vi "Build Support lvproj PPLs.vi"(8 "error in":errorcluster, 11 "custom device path":path) -> (0 "error out":errorcluster, 3 "custom device path out":path)   [LabVIEW 2020, in "Template Tool.lvlib"]
uses:
  Template Tool.lvlib
  Template Tool Global.vi
  <vilib>/AppBuilder/AB_API_Simple/NI_App_Builder_API.lvlib
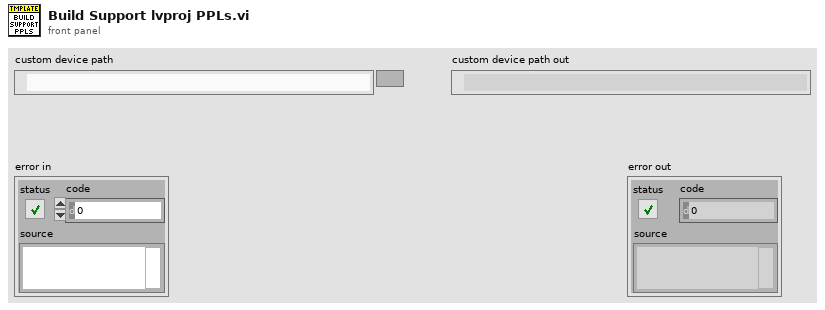
[diagram p1: front panel]
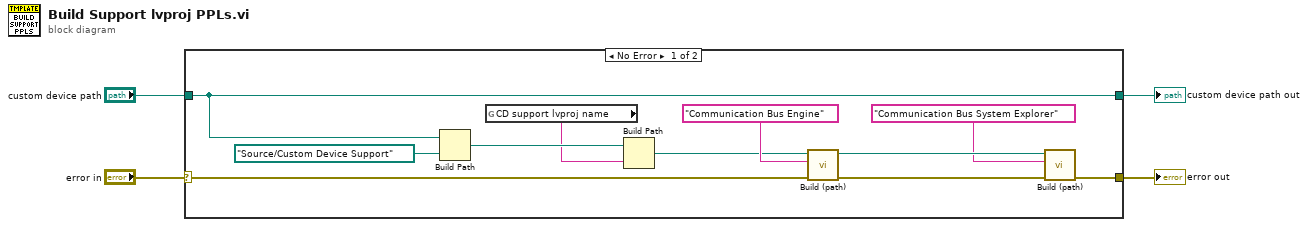
[diagram p0: block diagram]
diagram:
  n1 = case shown="No Error" "error in" {
    selector: "error in" -> [w11 w15]
    tunnel: "custom device path" -> [w12 w16]
    tunnel: [w6 w15] -> w4
    tunnel: [w12 w16] -> w1
    frame No Error {
      n2 = Build Path(base path=w12, name or relative path=path "Source/Custom Device Support") -> (appended path=w13:path)
      n3 = global read "Template Tool Global.vi" "CD support lvproj name"() -> (w5:string)
      n4 = Build Path(base path=w13, name or relative path=w5) -> (appended path=w9:path)
      n5 = call <vilib>:"Build (path).vi"("error in (no error)"=w11, "Name of build specification (if empty: build all)"="Communication Bus Engine" ("string"), "Path to project"=w9) -> ("error out"=w7:errorcluster)  [unwired: 7 in, 1 out]
      n6 = call <vilib>:"Build (path).vi"("error in (no error)"=w7, "Name of build specification (if empty: build all)"="Communication Bus System Explorer" ("string"), "Path to project"=w9) -> ("error out"=w6:errorcluster)  [unwired: 7 in, 1 out]
    }
    frame Error {
    }
  }
  "error out" <- w4
  "custom device path out" <- w1
